vi "4461 - Create AO waveforms.vi"(6 "sampling":T3={"Fs"=204789.0, "#s"=15753}, 8 "error in (no error)":errorcluster, 10 "reset signal":bool, 11 "AO":T1={"Ch"=[], "Amp (V)"=[0.1, 0.09, 0.08, 0.07, 0.06, 0.05, 0.04, 0.03], "DC (V)"=[0.0, 0.0, 0.0, 0.0, 0.0, 0.0, 0.0, 0.0], "f (Hz)"=[0.0, 0.0, 0.0, 0.0, 0.0, 0.0, 0.0, 0.0], "Phase (°)"=[13.0, 13.0, 13.0, 13.0, 13.0, 13.0, 13.0, 13.0], "Function"=[enum."Sine", enum."Sine", enum."Sine", enum."Sine", enum."Sine", enum."Sine", enum."Sine", enum."Sine"], "Sweep?"=[]} {"f (Hz)" min=0.001 max=10000.0 format="%.3g"; "Phase (°)" format="%.3g"; "DC (V)" format="%.3p"; "Amp (V)" min=0.0 max=10.0 format="%.3p"}) -> (0 "error out":errorcluster, 1 "phase out":dbl[](array[numeric]), 2 "AO Array":waveform(dbl)[](array[waveform]), 3 "AO out":T1={"Ch"=[], "Amp (V)"=[0.1, 0.09, 0.08, 0.07, 0.06, 0.05, 0.04, 0.03], "DC (V)"=[0.0, 0.0, 0.0, 0.0, 0.0, 0.0, 0.0, 0.0], "f (Hz)"=[0.0, 0.0, 0.0, 0.0, 0.0, 0.0, 0.0, 0.0], "Phase (°)"=[13.0, 13.0, 13.0, 13.0, 13.0, 13.0, 13.0, 13.0], "Function"=[enum."Sine", enum."Sine", enum."Sine", enum."Sine", enum."Sine", enum."Sine", enum."Sine", enum."Sine"], "Sweep?"=[]} {"f (Hz)" min=0.001 max=10000.0 format="%.3g"; "Phase (°)" format="%.3g"; "DC (V)" format="%.3p"; "Amp (V)" min=0.0 max=10.0 format="%.3p"})   [LabVIEW 2016, in "LockinDAQ.lvclass"]
uses:
  LockinDAQ.lvclass
  Typedefs/Sampling.ctl
  Typedefs/AO-cluster.ctl
  Typedefs/Function-enum.ctl
  <vilib>/measure/NI_MABase.lvlib
panel:
  out "Waveform Chart":dbl[][](graph)
  out "Waveform Graph":waveform(dbl)[](graph)
  out "Numeric":i32
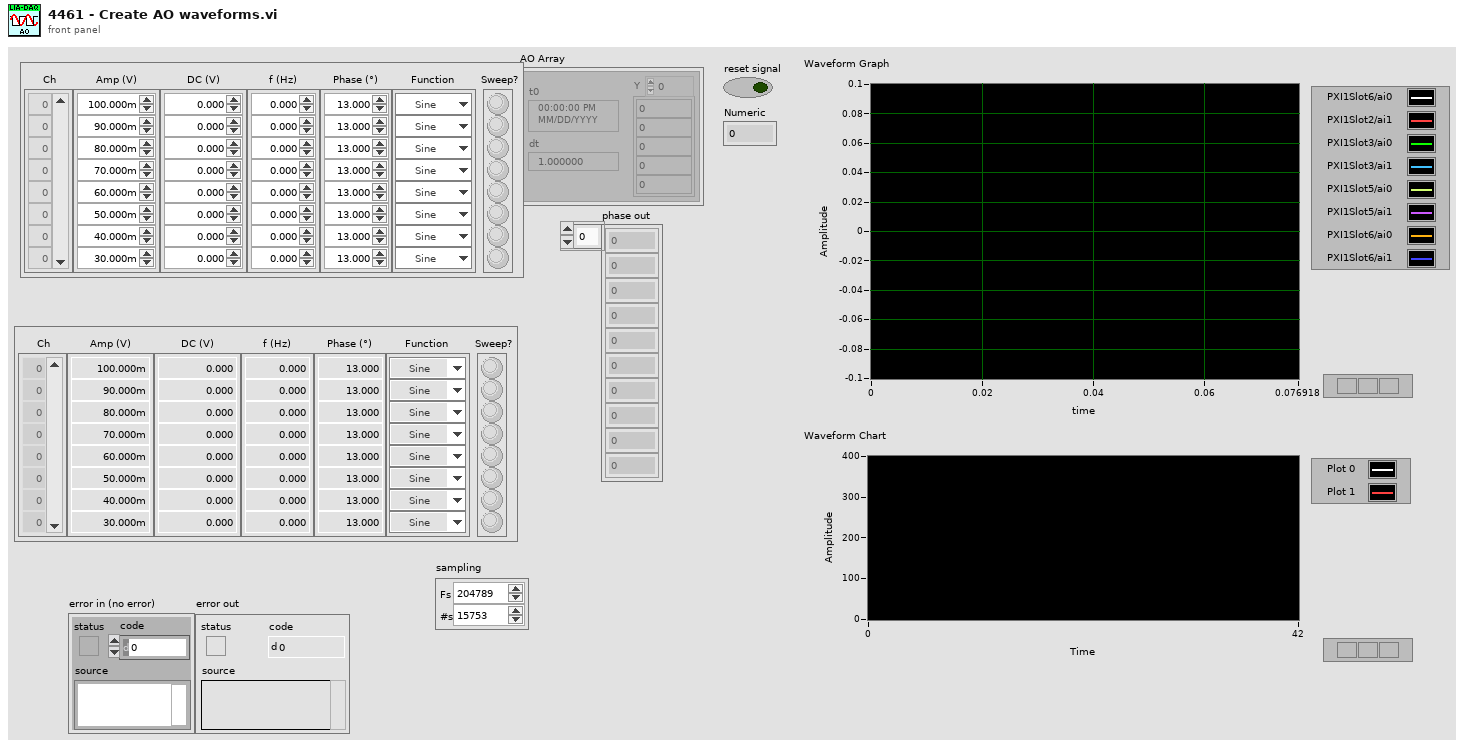
[diagram p1: front panel]
types:
  T1 = typedef "LockinDAQ.lvclass/AO-cluster.ctl" = cluster{"Ch":i32[], "Amp (V)":dbl[], "DC (V)":dbl[], "f (Hz)":dbl[], "Phase (°)":dbl[], "Function":T2[], "Sweep?":bool[]}
  T2 = typedef "LockinDAQ.lvclass/Function-enum.ctl" = enum16{"Sine", "Triangle", "Square", "Sawtooth"}
  T3 = typedef "LockinDAQ.lvclass/Sampling.ctl" = cluster{"Fs":dbl, "#s":i32}
  T4 = enum16{"Sine Wave", "Triangle Wave", "Square Wave", "Sawtooth Wave"}
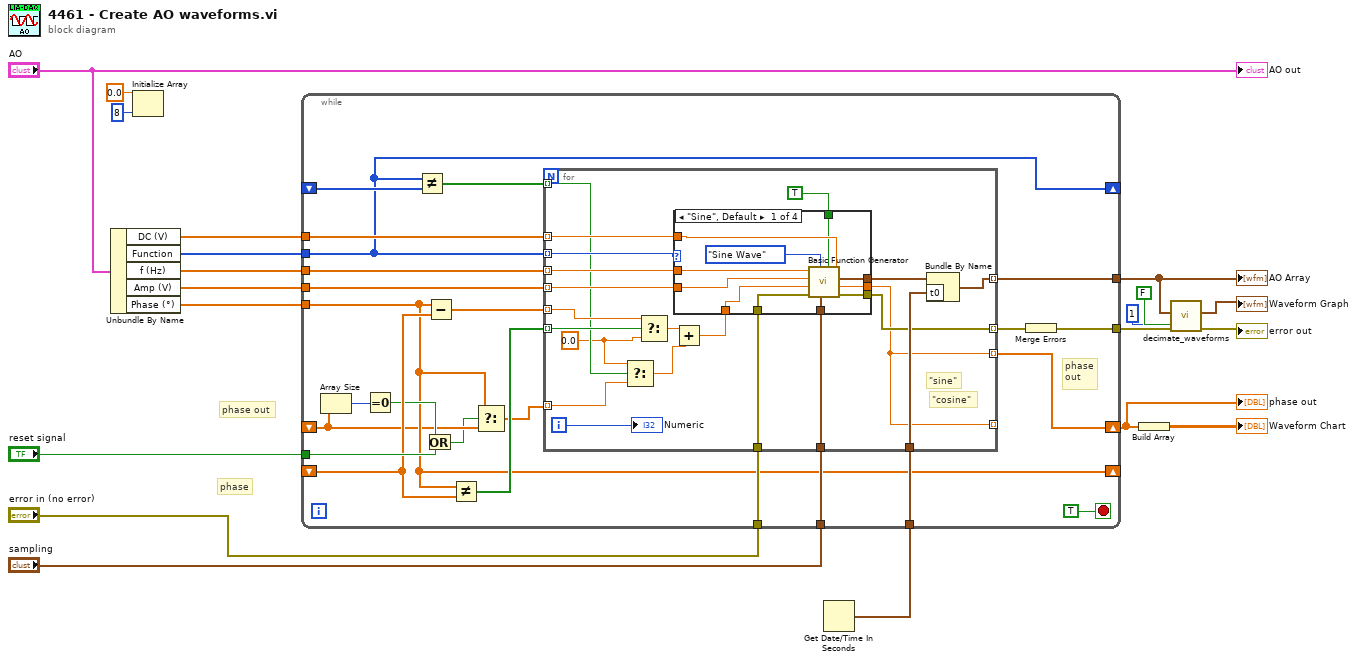
[diagram p0: block diagram]
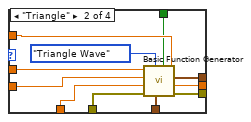
[diagram p2: hidden frame]
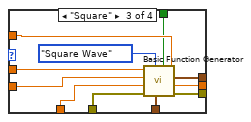
[diagram p3: hidden frame]
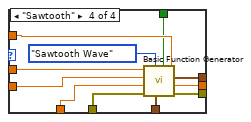
[diagram p4: hidden frame]
diagram:
  # "phase"
  # "phase out"
  n1 = Unbundle By Name("AO") -> ("DC (V)"=w19:dbl[], "Function"=w20:T2[], "f (Hz)"=w16:dbl[], "Amp (V)"=w17:dbl[], "Phase (°)"=w2:dbl[])
  n2 = Initialize Array(0.0 ("element"), 8 ("dimension size")) -> ()  [unwired: 1 out]
  n3 = Get Date/Time In Seconds() -> (seconds since 1Jan1904=w3:timestamp)
  n4 = while {
    tunnel: w20 -> [w26]
    tunnel: w19 -> [w44]
    tunnel: "sampling" -> [w43]
    tunnel: [w42] -> w12
    tunnel: w17 -> [w41]
    tunnel: w2 -> [w24]
    tunnel: w16 -> [w40]
    shift-right: [w24] -> _
    shift-left: _ -> [w29]
    shift-right: [w36] -> w7
    shift-left: _ -> [w22]
    tunnel: w3 -> [w35]
    tunnel: "reset signal" -> [w33]
    tunnel: "error in (no error)" -> [w32]
    tunnel: [w30] -> w10
    shift-right: [w26] -> _
    shift-left: _ -> [w27]
    stop <- TRUE stop-if-true
    # "phase\nout"
    n5 = Array Size(array=w22) -> (size(s)=w34:i32)
    n6 = Equal To 0?(x=w34) -> (x = 0?=w28:bool)
    n7 = Not Equal?(x=w26, y=w27) -> (x != y?=w25:bool[])
    n8 = Or(x=w28, y=w33) -> (x .or. y?=w21:bool)
    n9 = Subtract(x=w24, y=w29) -> (x-y=w37:dbl[])
    n10 = Not Equal?(x=w24, y=w29) -> (x != y?=w38:bool[])
    n11 = Select(t=w24, s=w21, f=w22) -> (s? t:f=w23:dbl[])
    n12 = for {
      tunnel: w26 -> [w49] mode=indexing
      tunnel: w40 -> [w65] mode=indexing
      tunnel: w41 -> [w52] mode=indexing
      tunnel: w44 -> [w64] mode=indexing
      tunnel: [w56] -> w42 mode=indexing
      tunnel: w43 -> [w50]
      tunnel: w38 -> [w60] mode=indexing
      tunnel: w37 -> [w61] mode=indexing
      tunnel: [w53] -> w36 mode=indexing
      tunnel: w35 -> [w59]
      tunnel: [w53] -> _ mode=indexing
      tunnel: w32 -> [w55]
      tunnel: [w54] -> w31 mode=indexing
      tunnel: w25 -> [w48] mode=indexing
      tunnel: w23 -> [w46] mode=indexing
      i -> [w58]
      w47 = 0.0 ("f")
      # "\"cosine\""
      # "\"sine\""
      n13 = Select(t=w47, s=w48, f=w46) -> (s? t:f=w45:dbl)
      n14 = Select(t=w61, s=w60, f=w47) -> (s? t:f=w62:dbl)
      n15 = Add(x=w62, y=w45) -> (x+y=w51:dbl)
      n16 = case shown="\"Sine\", Default" w49 {
        tunnel: w65 -> [w76 w87 w98 w109]
        tunnel: w64 -> [w75 w86 w97 w108]
        tunnel: [w74 w85 w96 w107] -> w63
        tunnel: TRUE ("reset signal") -> [w73 w84 w95 w106]
        tunnel: w55 -> [w72 w83 w94 w105]
        tunnel: [w71 w82 w93 w104] -> w54
        tunnel: [w70 w81 w92 w103] -> w53
        tunnel: w52 -> [w69 w80 w91 w102]
        tunnel: w51 -> [w68 w79 w90 w101]
        tunnel: w50 -> [w67 w78 w89 w100]
        frame "Sine", Default {
          n17 = call <vilib>:"Basic Function Generator.vi"("offset"=w75, "reset signal"=w73, "sampling info"=w67, "signal type"=T4."Sine Wave", "error in (no error)"=w72, "phase"=w68, "amplitude"=w69, "frequency"=w76) -> ("error out"=w71:errorcluster, "phase out"=w70:dbl, "signal out"=w74:waveform(dbl))  [unwired: 1 in]
        }
        frame "Triangle" {
          n18 = call <vilib>:"Basic Function Generator.vi"("offset"=w86, "reset signal"=w84, "sampling info"=w78, "signal type"=T4."Triangle Wave", "error in (no error)"=w83, "phase"=w79, "amplitude"=w80, "frequency"=w87) -> ("error out"=w82:errorcluster, "phase out"=w81:dbl, "signal out"=w85:waveform(dbl))  [unwired: 1 in]
        }
        frame "Square" {
          n19 = call <vilib>:"Basic Function Generator.vi"("offset"=w97, "reset signal"=w95, "sampling info"=w89, "signal type"=T4."Square Wave", "error in (no error)"=w94, "phase"=w90, "amplitude"=w91, "frequency"=w98) -> ("error out"=w93:errorcluster, "phase out"=w92:dbl, "signal out"=w96:waveform(dbl))  [unwired: 1 in]
        }
        frame "Sawtooth" {
          n20 = call <vilib>:"Basic Function Generator.vi"("offset"=w108, "reset signal"=w106, "sampling info"=w100, "signal type"=T4."Sawtooth Wave", "error in (no error)"=w105, "phase"=w101, "amplitude"=w102, "frequency"=w109) -> ("error out"=w104:errorcluster, "phase out"=w103:dbl, "signal out"=w107:waveform(dbl))  [unwired: 1 in]
        }
      }
      n21 = Bundle By Name(cluster=w63, "t0"=w59) -> (w56:waveform(dbl))
      "Numeric" <- w58
    }
    n22 = Merge Errors(w31) -> (w30:errorcluster)
  }
  "AO Array" <- w12
  "phase out" <- w7
  n23 = Build Array(w7) -> (→"Waveform Chart":dbl[][])
  n24 = call "decimate_waveforms.vi"("decimating factor"=1, "averaging"=FALSE, "error in (no error)"=w10, "WFM"=w12) -> ("error out"=→"error out":errorcluster, "WFM out"=→"Waveform Graph":waveform(dbl)[])  [unwired: 6 in]
  "AO out" <- "AO"
